vi "SparkLine_Create.vi"(0 "reference in":refnum<class "SparkLine.lvclass">, 2 "Override size":cluster{"Width":i16, "Height":i16}, 5 "error in (no error)":errorcluster) -> (14 "reference out":refnum<class "SparkLine.lvclass">, 19 "error out":errorcluster)   [LabVIEW 2019, in "SparkLine.lvclass"]
uses:
  SparkLine.lvclass
  C:/Users/Taylor.Hillegeist/OneDrive - Ultra/LabVIEW/Pgui2/Pgui_Obj_class/Pgui_Obj.lvclass
  Pgui_Obj_class/Pgui_Obj.lvclass
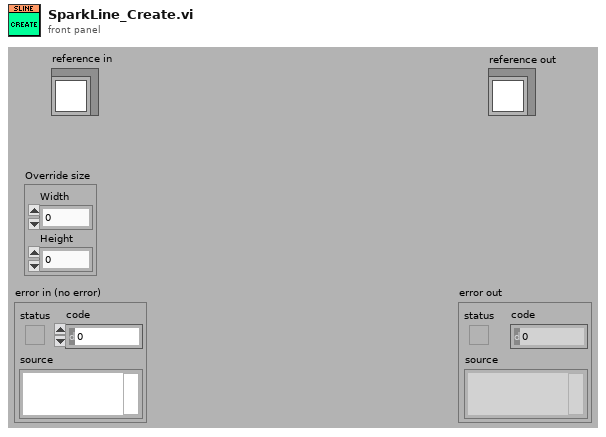
[diagram p1: front panel]
types:
  T1 = typedef "SparkLine.lvclass/ObjectAttributes.ctl" = cluster{"Override size":cluster{"Width":i16, "Height":i16}, "Data":dbl[]}
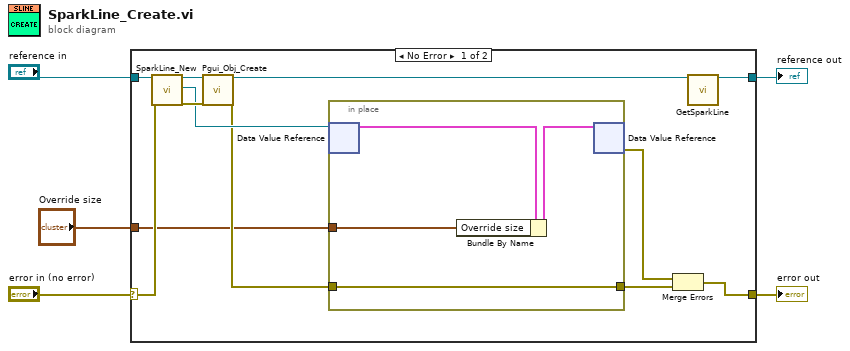
[diagram p0: block diagram]
diagram:
  n1 = case shown="No Error" "error in (no error)" {
    selector: "error in (no error)" -> [w16 w23]
    tunnel: [w14 w23] -> w4
    tunnel: "reference in" -> [w17 w22]
    tunnel: [w6 w22] -> w2
    tunnel: "Override size" -> [w8 _]
    frame No Error {
      n2 = call "SparkLine_New.vi"("reference in"=w17, "error in (no error)"=w16) -> ("reference out"=w13:refnum<class "SparkLine.lvclass">, "DVRRefOut"=w11:refnum<data-value>, "error out"=w12:errorcluster)  [unwired: 14 in, 1 out]
      n3 = call "Pgui_Obj_Create.vi"("reference in"=w13, "error in (no error)"=w12) -> ("reference out"=w7:refnum<class "SparkLine.lvclass">, "error out"=w10:errorcluster)  [unwired: 16 in]
      n4 = in-place {
        in-place-border: w10 -> [w19]
        in-place-border: [w19] -> w9
        in-place-border: w8 -> [w18]
        n5 = in-place-dvr #1(w11) -> (w20:T1)  [unwired: 1 out]
        n6 = Bundle By Name(cluster=w20, "Override size"=w18) -> (w21:T1)
        n7 = in-place-dvr #1(w21) -> (w15:errorcluster)  [unwired: 1 out]
      }
      n8 = Merge Errors(w15, w9) -> (w14:errorcluster)
      n9 = call-dynamic "GetSparkLine.vi"("reference in"=w7) -> ("reference out"=w6:refnum<class "SparkLine.lvclass">)  [unwired: 17 in, 1 out]
    }
    frame Error {
    }
  }
  "error out" <- w4
  "reference out" <- w2
